vi "7_convert temperature from Farenhiet to Celcius.vi"() -> ()   [LabVIEW 2018]
panel:
  out "Thermometer":dbl(slide) scale=0.0..100.0
  out "Temp in  C":dbl
  in  "Temp in F":dbl(slide) scale=0.0..100.0
  # "WAP to convert temperature from Farenhiet to Celcius"
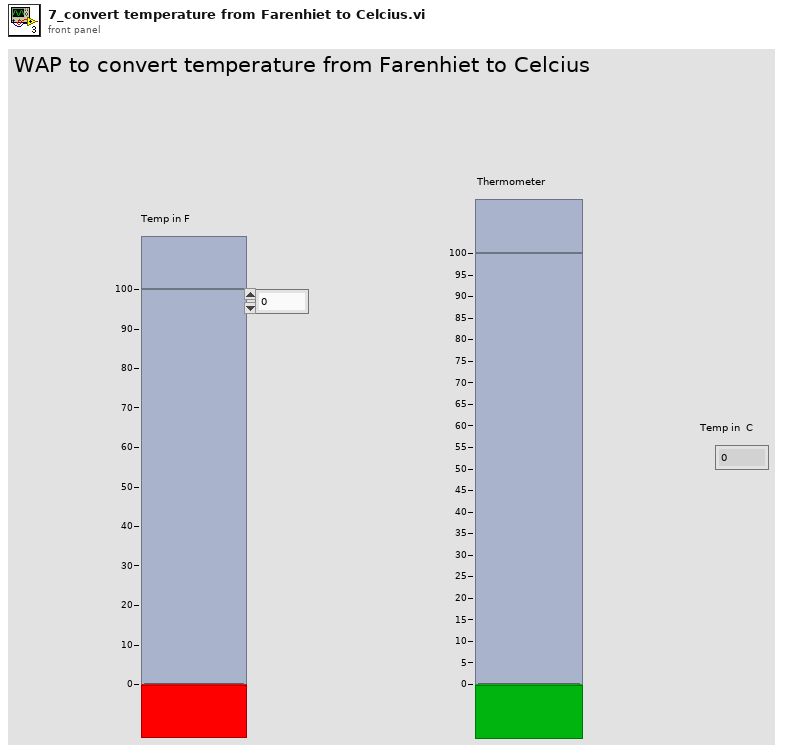
[diagram p1: front panel]
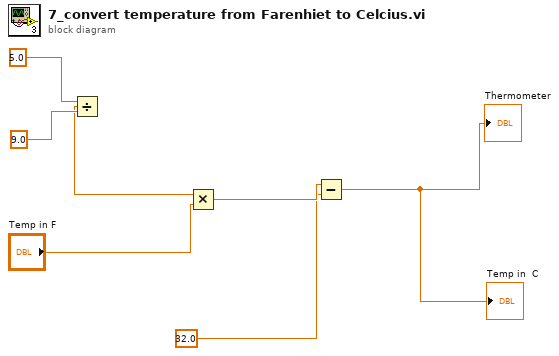
[diagram p0: block diagram]
diagram:
  n1 = Divide(x=5.0, y=9.0) -> (x/y=w5:dbl)
  n2 = Multiply(x=w5, y="Temp in F") -> (x*y=w3:dbl)
  n3 = Subtract(x=w3, y=32.0 ("x")) -> (x-y=→"Temp in  C" →"Thermometer":dbl)
